vi "PH_ImageStatistician.indicate Result.vi"(0 "i ref in":refnum<vi>, 5 "error in (no error)":errorcluster) -> (14 "i ref out":refnum<vi>, 19 "error out":errorcluster)   [LabVIEW 2014, in "PH_ImageStatistician.lvlib"]
doc: "This VI displays the results"
uses:
  PH_ImageStatistician.lvlib
  <vilib>/Analysis/NI_AALBase.lvlib
  <vilib>/Analysis/NI_AALPro.lvlib
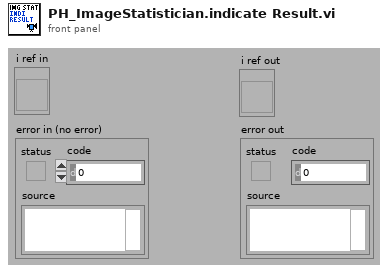
[diagram p1: front panel]
types:
  T1 = typedef "PH_ImageStatistician.lvlib/PH_ImageStatistician.i attribute.ctl" = cluster{"GUI Refs ":cluster{"Status":refnum<vi>, "Result Graph":refnum<vi>, "Mean Data 1":refnum<vi>, "Std Dev Data 1":refnum<vi>, "Mean Data 2":refnum<vi>, "Std Dev Data 2":refnum<vi>, "Mean Data 3":refnum<vi>, "Std Dev Data 3":refnum<vi>, "Dummy Mean":refnum<vi>, "Dummy Std Dev":refnum<vi>, "Export Data":refnum<vi>, "Data 1":refnum<vi>, "Data 2":refnum<vi>, "Data 3":refnum<vi>, "Stat or Trend":refnum<vi>, "Delete":refnum<vi>, "Operator":refnum<vi>, "Start":refnum<vi>}, "Operator":string, "Data":T2[], "Stat or Trend":bool, "Data 1":T3, "Data 2":T3, "Data 3":T3, "Start":bool, "Datasets strored":i32, "Dataarray Size":i32}
  T2 = typedef "PH_ImageStatistician.lvlib/PH_ImageStatistician.Statistician Data.ctl" = cluster{"Snapshot Time":dbl, "Maj FWHM":dbl, "Min FWHM":dbl, "Maj Fit Order":dbl, "Min Fit Order":dbl, "99% Diam Maj Trace":dbl, "99% Diam Min Trace":dbl, "Theta":dbl, "Delta":dbl, "Maj Diam":dbl, "Min Diam":dbl, "Azimuth Angle":dbl, "Azi Angle rel to major?":dbl, "Ellipticity":dbl, "CoG - X":dbl, "CoG - Y":dbl, "Energy":dbl, "Energy Cal - no mJ":dbl, "Lin Cal - no mm or mrad":dbl, "Lin Cal Factor":dbl}
  T3 = typedef "PH_ImageStatistician.lvlib/PH_ImageStatistician.select Data.ctl" = u16
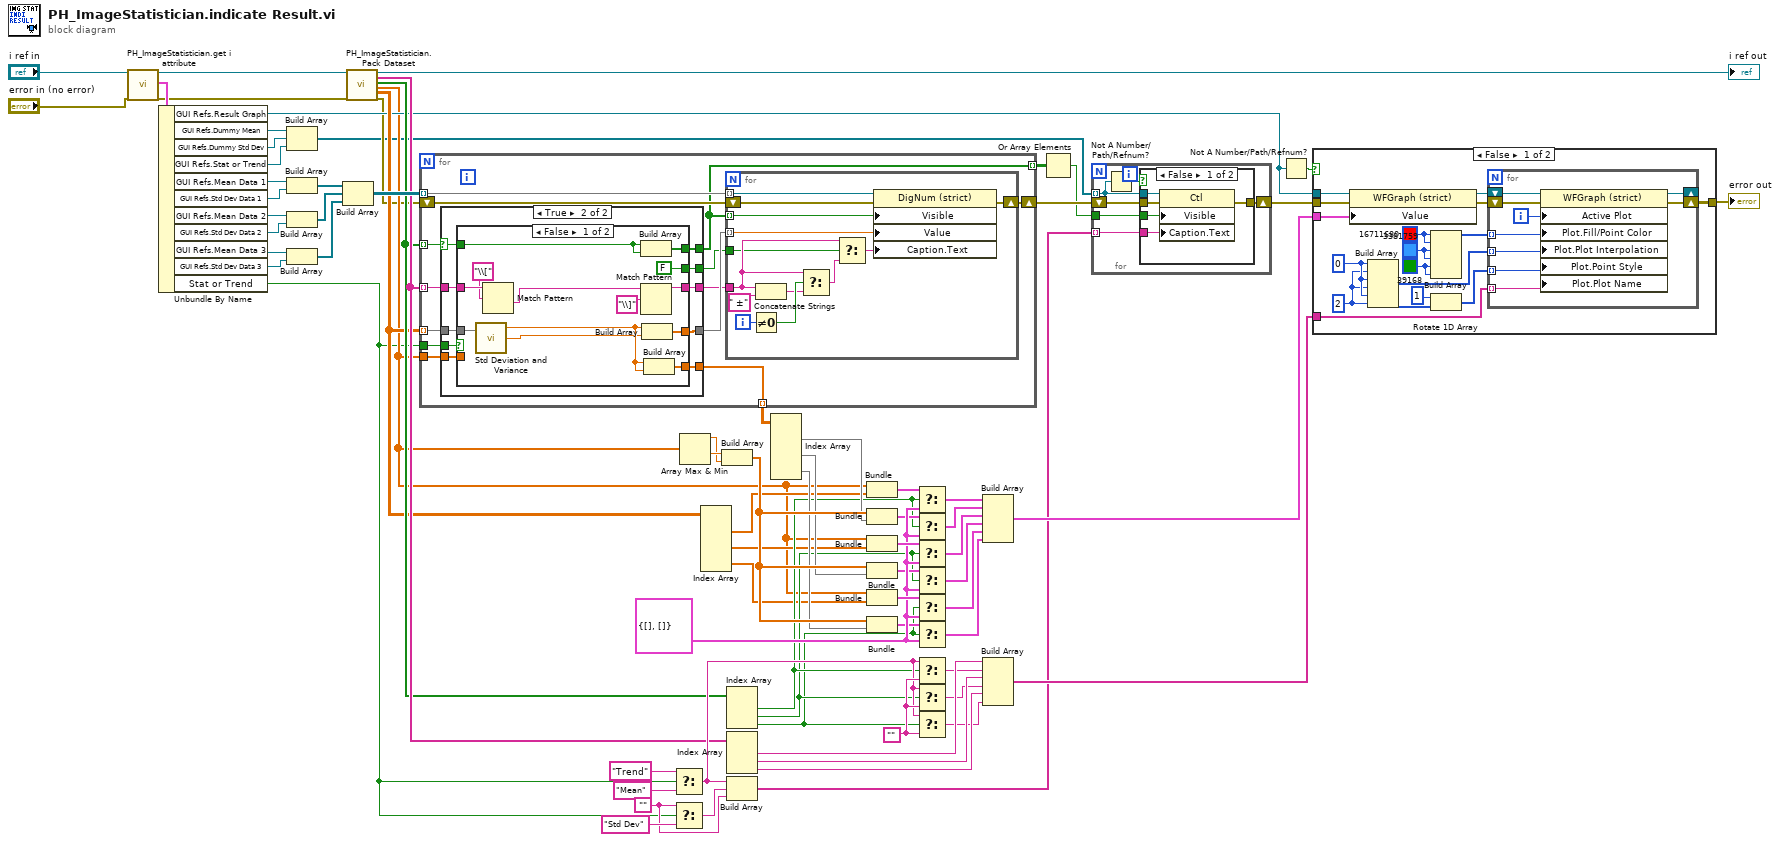
[diagram p0: block diagram]
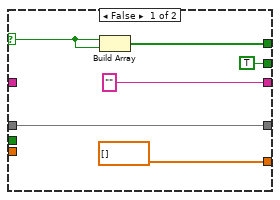
[diagram p4: hidden frame]
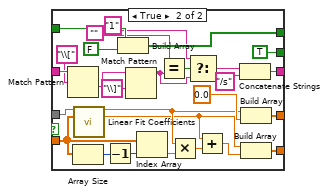
[diagram p5: hidden frame]
diagram:
  w37 = ""
  w44 = ""
  w54 = cluster{dbl[], dbl[]} {[], []} ("output cluster")
  n1 = call "PH_ImageStatistician.get i attribute.vi"("i ref in"="i ref in", "error in (no error)"="error in (no error)") -> ("i ref out"=w14:refnum<vi>, "i attribute"=w73:T1, "error out"=w8:errorcluster)  [unwired: 15 in]
  n2 = Unbundle By Name(w73) -> ("GUI Refs.Result Graph"=w17:refnum<vi>, "GUI Refs.Dummy Mean"=w6:refnum<vi>, "GUI Refs.Dummy Std Dev"=w5:refnum<vi>, "GUI Refs.Stat or Trend"=w4:refnum<vi>, "GUI Refs.Mean Data 1"=w64:refnum<vi>, "GUI Refs.Std Dev Data 1"=w63:refnum<vi>, "GUI Refs.Mean Data 2"=w62:refnum<vi>, "GUI Refs.Std Dev Data 2"=w12:refnum<vi>, "GUI Refs.Mean Data 3"=w65:refnum<vi>, "GUI Refs.Std Dev Data 3"=w66:refnum<vi>, "Stat or Trend"=w3:bool)
  n3 = Build Array(w6, w5, w4) -> (w9:refnum<vi>[])
  n4 = Build Array(w64, w63) -> (w61:refnum<vi>[])
  n5 = Build Array(w62, w12) -> (w60:refnum<vi>[])
  n6 = Build Array(w65, w66) -> (w59:refnum<vi>[])
  n7 = Build Array(w61, w60, w59) -> (w43:refnum<vi>[][])
  n8 = call "PH_ImageStatistician.Pack Dataset.vi"("i ref in"=w14, "error in"=w8) -> ("i ref out"=→"i ref out":refnum<vi>, "Dataset Legend"=w20:string[], "Dataset chosen?"=w19:bool[], "Timebase"=w16:dbl[], "Dataset"=w18:dbl[][], "error out"=w15:errorcluster)  [unwired: 12 in]
  n9 = for {
    tunnel: w18 -> [w88] mode=indexing
    tunnel: w43 -> [w87] mode=indexing
    shift-right: [w85] -> w11
    shift-left: w15 -> [w84]
    tunnel: w19 -> [w81] mode=indexing
    tunnel: w20 -> [w83] mode=indexing
    tunnel: [w79] -> w55 mode=indexing
    tunnel: w3 -> [w80]
    tunnel: w16 -> [w78]
    tunnel: [w77] -> w2 mode=indexing
    n10 = case shown="True" w81 {
      selector: w81 -> [w92 w100]
      tunnel: w88 -> [w93 w104]
      tunnel: [w93 w103] -> w86
      tunnel: w83 -> [_ w102]
      tunnel: ["" ("Data Legend") w101] -> w82
      tunnel: [w91 w99] -> w77
      tunnel: w80 -> [_ w98]
      tunnel: [dbl[] [] w97] -> w79
      tunnel: w78 -> [_ w96]
      tunnel: [TRUE w95] -> w76
      frame False {
        n11 = Build Array(w92, w92) -> (w91:bool[])
      }
      frame True {
        n12 = case shown="False" w98 {
          tunnel: w104 -> [w109 w128]
          tunnel: [w117 w144] -> w103
          tunnel: w102 -> [w116 w143]
          tunnel: [w106 w130] -> w101
          tunnel: w100 -> [w112 w139]
          tunnel: [w111 w138] -> w99
          tunnel: [w110 w127] -> w97
          tunnel: w96 -> [_ w126]
          tunnel: [FALSE TRUE] -> w95
          frame False {
            n13 = call <vilib>:"Std Deviation and Variance.vi"("X"=w109) -> ("mean"=w108:dbl, "standard deviation"=w107:dbl)  [unwired: 1 in, 1 out]
            n14 = Match Pattern(string=w116, regular expression="\\[") -> (after substring=w114:string)  [unwired: 1 in, 3 out]
            n15 = Build Array(w112, w112) -> (w111:bool[])
            n16 = Match Pattern(string=w114, regular expression="\\]") -> (before substring=w106:string)  [unwired: 1 in, 3 out]
            n17 = Build Array(w108, w107) -> (w117:dbl[])
            n18 = Build Array(w108, w108) -> (w110:dbl[])
          }
          frame True {
            n19 = Match Pattern(string=w143, regular expression="\\[") -> (after substring=w141:string)  [unwired: 1 in, 3 out]
            n20 = Array Size(array=w126) -> (size(s)=w125:i32)
            n21 = call <vilib>:"Linear Fit Coefficients.vi"("Y"=w128, "X"=w126) -> ("slope"=w122:dbl, "intercept"=w120:dbl)  [unwired: 11 in, 1 out]
            n22 = Decrement(x=w125) -> (x-1=w124:i32)
            n23 = Build Array(w139, FALSE ("element")) -> (w138:bool[])
            n24 = Match Pattern(string=w141, regular expression="\\]") -> (before substring=w133:string)  [unwired: 1 in, 3 out]
            n25 = Index Array(array=w126, index=w124) -> (element=w123:dbl)
            n26 = Equal?(x="", y=w133) -> (x = y?=w134:bool)
            n27 = Multiply(x=w122, y=w123) -> (x*y=w121:dbl)
            n28 = Select(t="1" ("regular expression"), s=w134, f=w133) -> (s? t:f=w131:string)
            n29 = Add(x=w120, y=w121) -> (x+y=w119:dbl)
            n30 = Concatenate Strings(w131, "/s" ("regular expression")) -> (w130:string)
            n31 = Build Array(w122, 0.0 ("element")) -> (w144:dbl[])
            n32 = Build Array(w120, w119) -> (w127:dbl[])
          }
        }
      }
    }
    n33 = for {
      tunnel: w87 -> [w157] mode=indexing
      tunnel: w86 -> [w156] mode=indexing
      shift-right: [w154] -> w85
      shift-left: w84 -> [w155]
      tunnel: w77 -> [w153] mode=indexing
      tunnel: w82 -> [w147]
      tunnel: w76 -> [w145]
      i -> [w152]
      n34 = Not Equal To 0?(x=w152) -> (x != 0?=w151:bool)
      n35 = Concatenate Strings(w147, " ±") -> (w149:string)
      n36 = Select(t=w147, s=w151, f=w149) -> (s? t:f=w148:string)
      n37 = Select(t=w147, s=w145, f=w148) -> (s? t:f=w146:string)
      n38 = property class="DigNum (strict)"(reference=w157, error in=w155, "Visible"=w153, "Value"=w156, "Caption.Text"=w146) -> (error out=w154:errorcluster)  [unwired: 1 out]
    }
  }
  n39 = Select(t="Trend" ("Plot.Plot Name"), s=w3, f="Mean") -> (s? t:f=w38:string)
  n40 = Select(t=w37, s=w3, f="Std Dev") -> (s? t:f=w42:string)
  n41 = Array Max & Min(array=w16) -> (max value=w57:dbl, min value=w58:dbl)  [unwired: 2 out]
  n42 = Index Array(array=w18) -> (element #1=w25:dbl[], element #2=w24:dbl[], element #3=w21:dbl[])  [unwired: 6 in]
  n43 = Build Array(w58, w57) -> (w56:dbl[])
  n44 = Index Array(array=w19) -> (element #1=w28:bool, element #2=w27:bool, element #3=w26:bool)  [unwired: 3 in]
  n45 = Index Array(array=w20) -> (element #1=w36:string, element #2=w35:string, element #3=w34:string)  [unwired: 3 in]
  n46 = Build Array(w38, w42, w37) -> (w7:string[])
  n47 = Index Array(array=w55) -> (element #1=w47:dbl[], element #2=w46:dbl[], element #3=w45:dbl[])  [unwired: 6 in]
  n48 = Bundle("Timebase"=w16, "Dataset"=w25) -> (w72:cluster{"Timebase":dbl[], "Dataset":dbl[]})  [unwired: 1 in]
  n49 = Bundle(w56, w47) -> (w51:cluster{dbl[], dbl[]})  [unwired: 1 in]
  n50 = Bundle("Timebase"=w16, "Dataset"=w24) -> (w70:cluster{"Timebase":dbl[], "Dataset":dbl[]})  [unwired: 1 in]
  n51 = Bundle(w56, w46) -> (w52:cluster{dbl[], dbl[]})  [unwired: 1 in]
  n52 = Bundle("Timebase"=w16, "Dataset"=w21) -> (w69:cluster{"Timebase":dbl[], "Dataset":dbl[]})  [unwired: 1 in]
  n53 = Bundle(w56, w45) -> (w53:cluster{dbl[], dbl[]})  [unwired: 1 in]
  n54 = Select(t=w72, s=w28, f=w54) -> (s? t:f=w71:cluster{"Timebase":dbl[], "Dataset":dbl[]})
  n55 = Select(t=w51, s=w28, f=w54) -> (s? t:f=w50:cluster{dbl[], dbl[]})
  n56 = Select(t=w70, s=w27, f=w54) -> (s? t:f=w68:cluster{"Timebase":dbl[], "Dataset":dbl[]})
  n57 = Select(t=w52, s=w27, f=w54) -> (s? t:f=w49:cluster{dbl[], dbl[]})
  n58 = Select(t=w69, s=w26, f=w54) -> (s? t:f=w67:cluster{"Timebase":dbl[], "Dataset":dbl[]})
  n59 = Select(t=w53, s=w26, f=w54) -> (s? t:f=w48:cluster{dbl[], dbl[]})
  n60 = Select(t=w38, s=w28, f=w44) -> (s? t:f=w33:string)
  n61 = Select(t=w38, s=w27, f=w44) -> (s? t:f=w32:string)
  n62 = Select(t=w38, s=w26, f=w44) -> (s? t:f=w31:string)
  n63 = Build Array(w71, w50, w68, w49, w67, w48) -> (w29:cluster{"Timebase":dbl[], "Dataset":dbl[]}[])
  n64 = Build Array(w36, w33, w35, w32, w34, w31) -> (w30:string[])
  n65 = Or Array Elements(Boolean array=w2) -> (logical OR=w1:bool)
  n66 = for {
    tunnel: w9 -> [w159] mode=indexing
    shift-right: [w162] -> w10
    shift-left: w11 -> [w163]
    tunnel: w7 -> [w161] mode=indexing
    tunnel: w1 -> [w158]
    n67 = Not A Number/Path/Refnum?(number/path/refnum=w159) -> (NaN/Path/Refnum?=w160:bool)
    n68 = case shown="False" w160 {
      tunnel: w159 -> [w168 _]
      tunnel: w163 -> [w167 w169]
      tunnel: [w166 w169] -> w162
      tunnel: w161 -> [w165 _]
      tunnel: w158 -> [w164 _]
      frame False {
        n69 = property class="Ctl"(reference=w168, error in=w167, "Visible"=w164, "Caption.Text"=w165) -> (error out=w166:errorcluster)  [unwired: 1 out]
      }
      frame True {
      }
    }
  }
  n70 = Not A Number/Path/Refnum?(number/path/refnum=w17) -> (NaN/Path/Refnum?=w22:bool)
  n71 = case shown="False" w22 {
    tunnel: w30 -> [w176 _]
    tunnel: w29 -> [w175 _]
    tunnel: w17 -> [w174 _]
    tunnel: w10 -> [w172 w195]
    tunnel: [w170 w195] -> w23
    frame False {
      w180 = u8 2 ("Plot.Plot Interpolation")
      w181 = u8 0 ("Plot.Plot Interpolation")
      w184 = u32 39168 ("Color Box")
      w183 = u32 3381759 ("Color Box")
      w185 = u32 16711680 ("Color Box")
      n72 = property class="WFGraph (strict)"(reference=w174, error in=w172, "Value"=w175) -> (reference out=w173:refnum<vi>, error out=w171:errorcluster)
      n73 = Build Array(w181, w180, w181, w180, w181, w180) -> (w179:u8[])
      n74 = Build Array(w185, w185, w183, w183, w184, w184) -> (w182:u32[])
      n75 = Rotate 1D Array(1:w179, 2:1 ("n")) -> (0:w177:u8[])
      n76 = for {
        shift-right: [w194] -> _
        shift-left: w173 -> [w193]
        shift-right: [w192] -> w170
        shift-left: w171 -> [w191]
        tunnel: w182 -> [w189] mode=indexing
        tunnel: w179 -> [w188] mode=indexing
        tunnel: w177 -> [w187] mode=indexing
        tunnel: w176 -> [w186] mode=indexing
        i -> [w190]
        n77 = property class="WFGraph (strict)"(reference=w193, error in=w191, "Active Plot"=w190, "Plot.Fill/Point Color"=w189, "Plot.Plot Interpolation"=w188, "Plot.Point Style"=w187, "Plot.Plot Name"=w186) -> (reference out=w194:refnum<vi>, error out=w192:errorcluster)
      }
    }
    frame True {
    }
  }
  "error out" <- w23
